vi "Logger.File.Read.Serials2.vi"(8 "error in":errorcluster, 11 "file ref in":refnum<k34>) -> (0 "error out":errorcluster, 2 "Data":T2[](array[typedef]), 3 "file ref out":refnum<k34>)   [LabVIEW 2016]
uses:
  Logger.File.Serials.ctl
  Sequence/Sequence.Step.Status.ctl
panel:
  in  "Status":T1
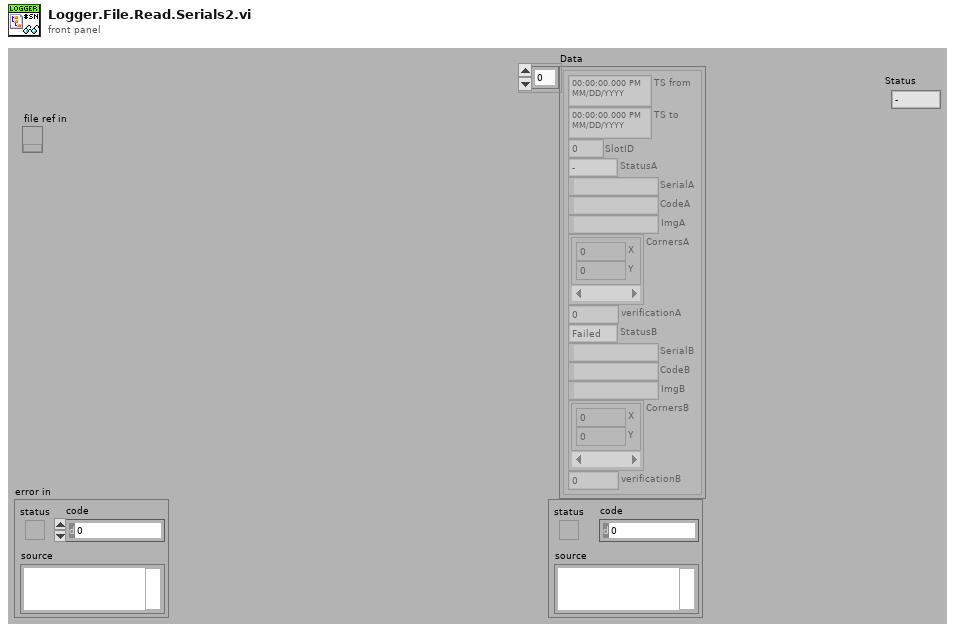
[diagram p1: front panel]
types:
  T1 = typedef "Sequence.Step.Status.ctl" = enum16{"-", "Pending", "Running", "Skipped", "Passed", "Failed", "Done", "Error", "Aborted", "Stopped"}
  T2 = typedef "Logger.File.Serials.ctl" = cluster{"TS from":timestamp, "TS to":timestamp, "SlotID":u8, "StatusA":T1, "SerialA":string, "CodeA":string, "ImgA":string, "CornersA":cluster{"X":i32, "Y":i32}[], "verificationA":u8, "StatusB":T1, "SerialB":string, "CodeB":string, "ImgB":string, "CornersB":cluster{"X":i32, "Y":i32}[], "verificationB":u8}
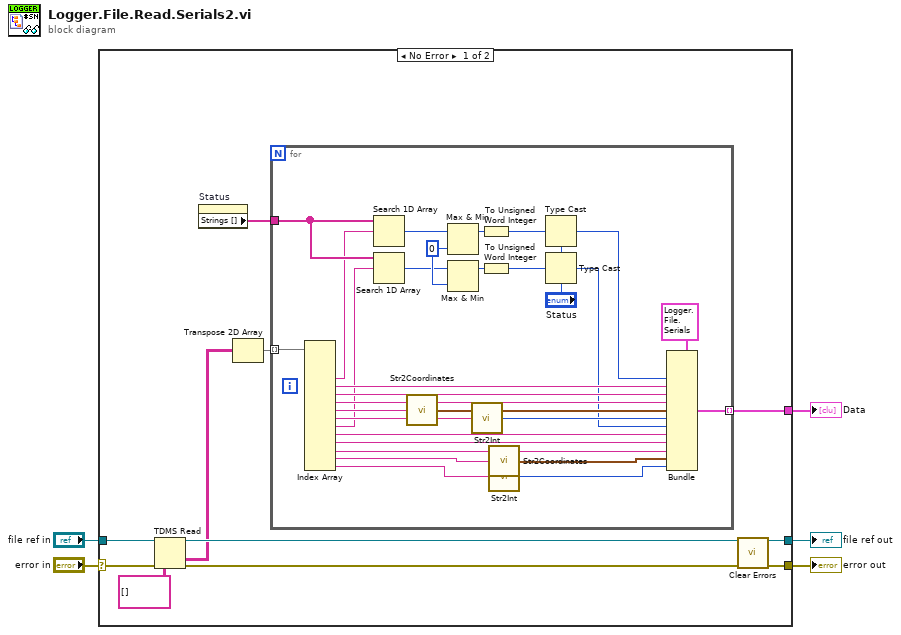
[diagram p0: block diagram]
diagram:
  n1 = case shown="No Error" "error in" {
    selector: "error in" -> [w13 w47]
    tunnel: [w12 w47] -> w5
    tunnel: "file ref in" -> [w14 w46]
    tunnel: [w9 w46] -> w4
    tunnel: [w11 _] -> w1
    frame No Error {
      n2 = TDMS Read(0:w14, 11:w13, 12:string[][] [] ("appended array")) -> (4:w9:refnum<k34>, 10:w8:string[][], 15:w15:errorcluster)  [unwired: 5 in, 3 out]
      n3 = property on="Status" class="Enum (strict)"() -> ("Strings []"=w6:string[])  [unwired: 2 in, 2 out]
      n4 = Transpose 2D Array(2D array=w8) -> (transposed array=w7:string[][])
      n5 = for {
        tunnel: w7 -> [w44] mode=indexing
        tunnel: [w45] -> w11 mode=indexing
        tunnel: w6 -> [w20]
        w28 = 0 ("y")
        n6 = Index Array(array=w44) -> (element #3=w19:string, element #4=w29:string, element #5=w42:string, element #6=w31:string, element #7=w41:string, element #8=w33:string, element #9=w18:string, element #10=w30:string, element #11=w38:string, element #12=w32:string, element #13=w36:string, element #14=w35:string)  [unwired: 14 in, 2 out]
        n7 = Search 1D Array(1D array=w20, element=w19) -> (index of element=w21:i32)  [unwired: 1 in]
        n8 = Search 1D Array(1D array=w20, element=w18) -> (index of element=w26:i32)  [unwired: 1 in]
        n9 = call "Str2Coordinates.vi"("String"=w41) -> ("Coordinates"=w40:cluster{"X":dbl, "Y":dbl}[])  [unwired: 1 in]
        n10 = Max & Min(x=w21, y=w28) -> (max(x,y)=w22:i32)  [unwired: 1 out]
        n11 = Max & Min(x=w26, y=w28) -> (max(x,y)=w25:i32)  [unwired: 1 out]
        n12 = call "Str2Int.vi"("string"=w33) -> ("Numeric"=w39:i32)
        n13 = To Unsigned Word Integer(number=w22) -> (unsigned 16bit integer=w23:u16)
        n14 = To Unsigned Word Integer(number=w25) -> (unsigned 16bit integer=w24:u16)
        n15 = call "Str2Coordinates.vi"("String"=w36) -> ("Coordinates"=w37:cluster{"X":dbl, "Y":dbl}[])  [unwired: 1 in]
        n16 = call "Str2Int.vi"("string"=w35) -> ("Numeric"=w34:i32)
        n17 = Type Cast(type="Status", x=w23) -> (*(type *) &x=w16:T1)
        n18 = Type Cast(type="Status", x=w24) -> (*(type *) &x=w17:T1)
        n19 = Bundle(cluster=T2 {"TS from"=timestamp(0 s since 1904-01-01), "TS to"=timestamp(0 s since 1904-01-01), "SlotID"=0, "StatusA"=enum."-", "SerialA"="", "CodeA"="", "ImgA"="", "CornersA"=[], "verificationA"=0, "StatusB"=enum."Failed", "SerialB"="", "CodeB"="", "ImgB"="", "CornersB"=[], "verificationB"=0} ("SerialData"), "StatusA"=w16, "SerialA"=w29, "CodeA"=w42, "ImgA"=w31, "CornersA"=w40, "verificationA"=w39, "StatusB"=w17, "SerialB"=w30, "CodeB"=w38, "ImgB"=w32, "CornersB"=w37, "verificationB"=w34) -> (w45:T2)  [unwired: 3 in]
      }
      n20 = call <vilib>:"Clear Errors.vi"("error in (no error)"=w15) -> ("error out"=w12:errorcluster)  [unwired: 5 in, 1 out]
    }
    frame Error {
    }
  }
  "error out" <- w5
  "file ref out" <- w4
  "Data" <- w1
